vi "FTW-Example-SLASD-Disconnect.vi"(0 "FTW-Example-SLASD In":refnum<class "FTW-Example-SLASD.lvclass">, 11 "error in (no error)":errorcluster) -> (15 "error out":errorcluster)   [LabVIEW 2013, in "FTW-Example-SLASD.lvclass"]
uses:
  FTW-Example-SLASD.lvclass
  FTW-Example-SLASD.lvclass/FTW-Example-SLASD.ctl
  Actor/src/Subscription/FTW-Subscription.lvclass
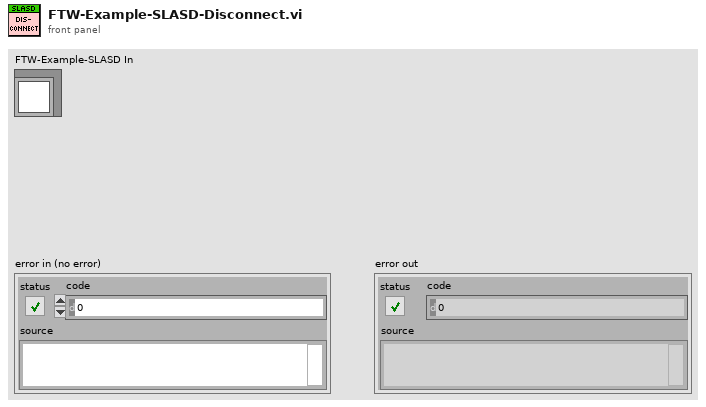
[diagram p1: front panel]
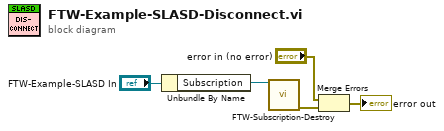
[diagram p0: block diagram]
diagram:
  n1 = Unbundle By Name("FTW-Example-SLASD In") -> ("Subscription"=w2:refnum<class "FTW-Subscription.lvclass">)
  n2 = call "FTW-Subscription-Destroy.vi"("FTW-Subscription In"=w2) -> ("error out"=w1:errorcluster)  [unwired: 14 in]
  n3 = Merge Errors("error in (no error)", w1) -> (→"error out":errorcluster)
